vi "COD主界面.vi"() -> ()   [LabVIEW 2016]
uses:
  <vilib>/Utility/miscctls.llb/LVPointTypeDef.ctl
  <vilib>/Plasmionique/MB Master/MB_Master_Serial/MB_Master_Serial.lvclass
  F:/Program Files/National Instruments/LabVIEW 2016/vi.lib/Plasmionique/MB Master/MB_Master/MB_Master.lvclass
  <vilib>/Plasmionique/MB Master/MB Master.lvlib
panel:
  out "COD浓度（mg/L)":dbl
  out "模式选择":u16(ring) items=["COD水样测量", "COD标样核查", "COD加标回收", "COD平行样", "COD校零", "COD校标"]
  out "table 输入":string
  out "columns":string[](array[string])
  in  "保存":bool
  out "data":T1
  out "多列列表框":i32(listbox)
  in  "温度 2":dbl
  in  "恒温时间":dbl
  in  "浓度":dbl
  in  "修正系数":dbl
  in  "基本量程":enum16{"10mL", "20mL"}(ring)
  in  "水样":dbl
  in  "蒸馏水":dbl
  in  "标液":dbl
  in  "质控样":dbl
  in  "加标回收":dbl
  in  "草酸钠":dbl
  in  "高锰酸钾":dbl
  in  "硫酸":dbl
  in  "关闭":bool
  in  "零点泵计量数 2":dbl
  in  "标度泵计量数 2":dbl
  in  "标样浓度 2":dbl
  in  "unit ID":u8=1 caption="单元ID"
  out "泵1计数":dbl
  out "泵2计数":dbl
  out "泵3计数":dbl
  out "泵4计数":dbl
  out "标度滴定值":dbl
  out "零点滴定值":dbl
  in  "启动":bool
  in  "故障清除":bool
  out "排液阀故障":bool
  out "进水样超量程":bool
  out "模式（受控）":u16
  out "ORP显示":dbl
  out "温度":dbl
  out "标样核查标记":bool
  out "平行样测量":bool
  out "加标回收测量":bool
  out "质控样测量":bool
  out "待机":bool
  out "校标错误":bool
  out "校零错误":bool
  out "测量错误":bool
  out "草酸钠报警":bool
  out "高锰酸钾报警":bool
  out "加热故障":bool
  out "温控器故障":bool
  out "ORP故障":bool
  out "排液标记":bool
  out "故障标记":bool
  out "校标标记":bool
  out "校零标记":bool
  out "通讯状态":bool
  out "水样测量":bool
  in  "参数配置":bool
  in  "VISA resource name":refnum<visa-resource-name> caption="VISA资源名称"
  in  "停止 2":bool
  in  "停止":bool
  in  "单步启动":bool
  # "mV"
  # "℃"
  # "水样~加标回收"
  # "高锰酸钾"
  # "草酸钠"
  # "硫酸"
  # "基本参数设置"
  # "泵计量参数设置"
  # "校零校标结果"
  # "加热恒温温度（℃）："
  # "水样："
  # "高锰酸钾："
  # "校零结果："
  # "校零滴定值："
  # "恒温时间（分钟）："
  # "蒸馏水："
  # "草酸钠："
  # "校标结果："
  # "标度滴定值："
  # "零点泵计量值："
  # "标准液浓度（mg/L）："
  # "标液："
  # "硫酸："
  # "标度泵计量值："
  # "修正系数："
  # "质控样："
  # "标样浓度："
  # "加标回收样："
  # "基本量程（20mL可选）："
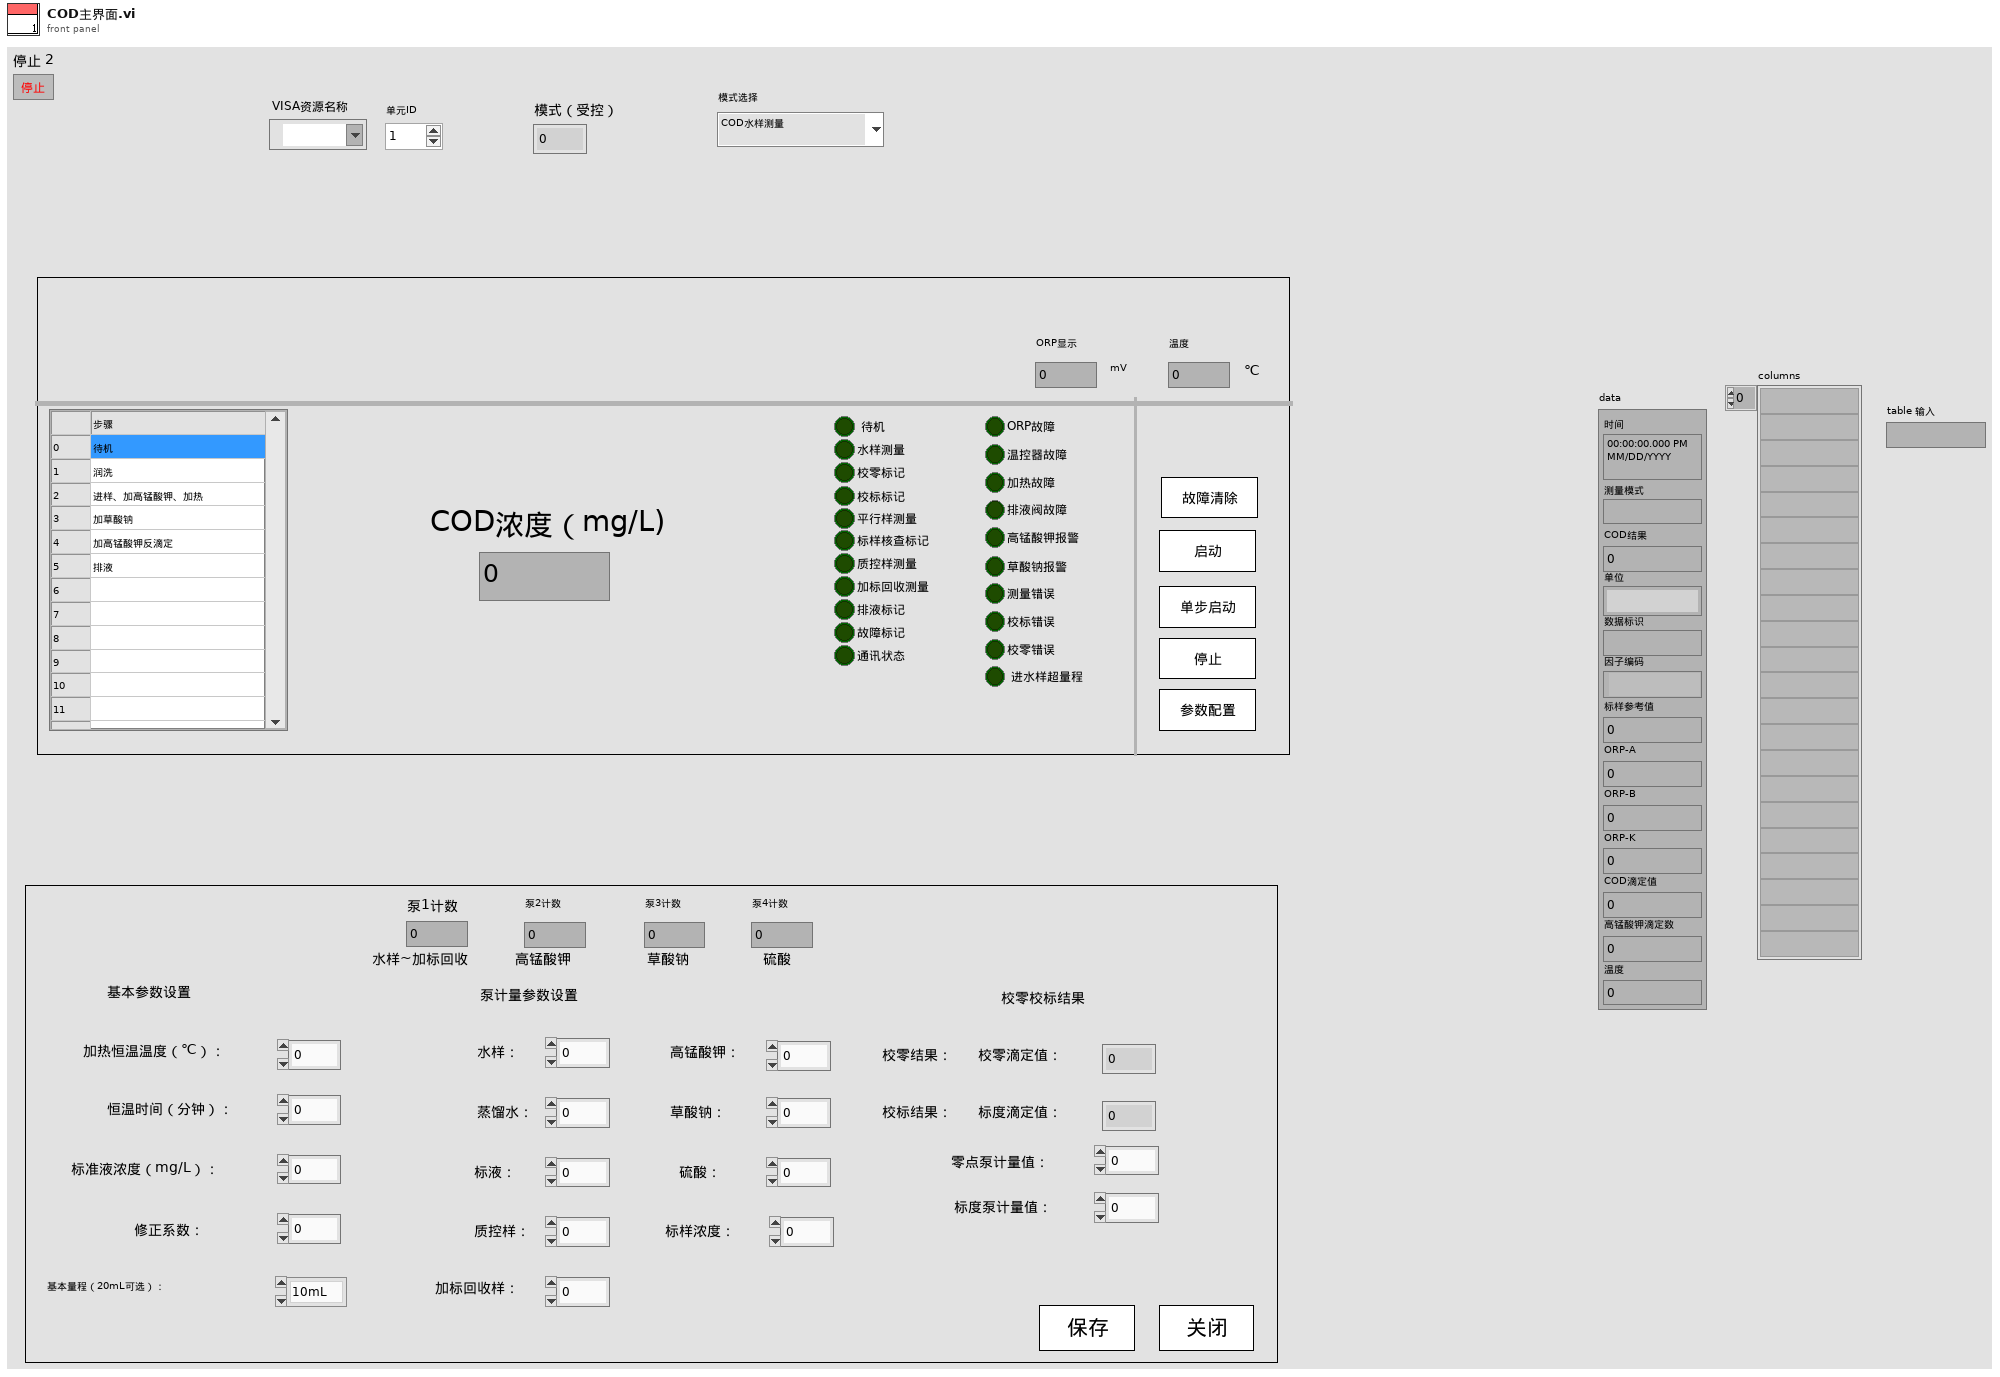
[diagram p1: front panel]
types:
  T1 = cluster{"时间":timestamp, "测量模式":string, "COD结果":sgl, "单位":string, "数据标识":string, "因子编码":string, "标样参考值":sgl, "ORP-A":sgl, "ORP-B":sgl, "ORP-K":sgl, "COD滴定值":sgl, "高锰酸钾滴定数":sgl, "温度":sgl}
  T2 = cluster{"baud rate (bps)":u32, "stop bits":u16, "parity":u16, "flow control":u16, "timeout":u32, "retries":i32}
  T3 = typedef "LVPointTypeDef.ctl" = cluster{"Horizontal":i16, "Vertical":i16}
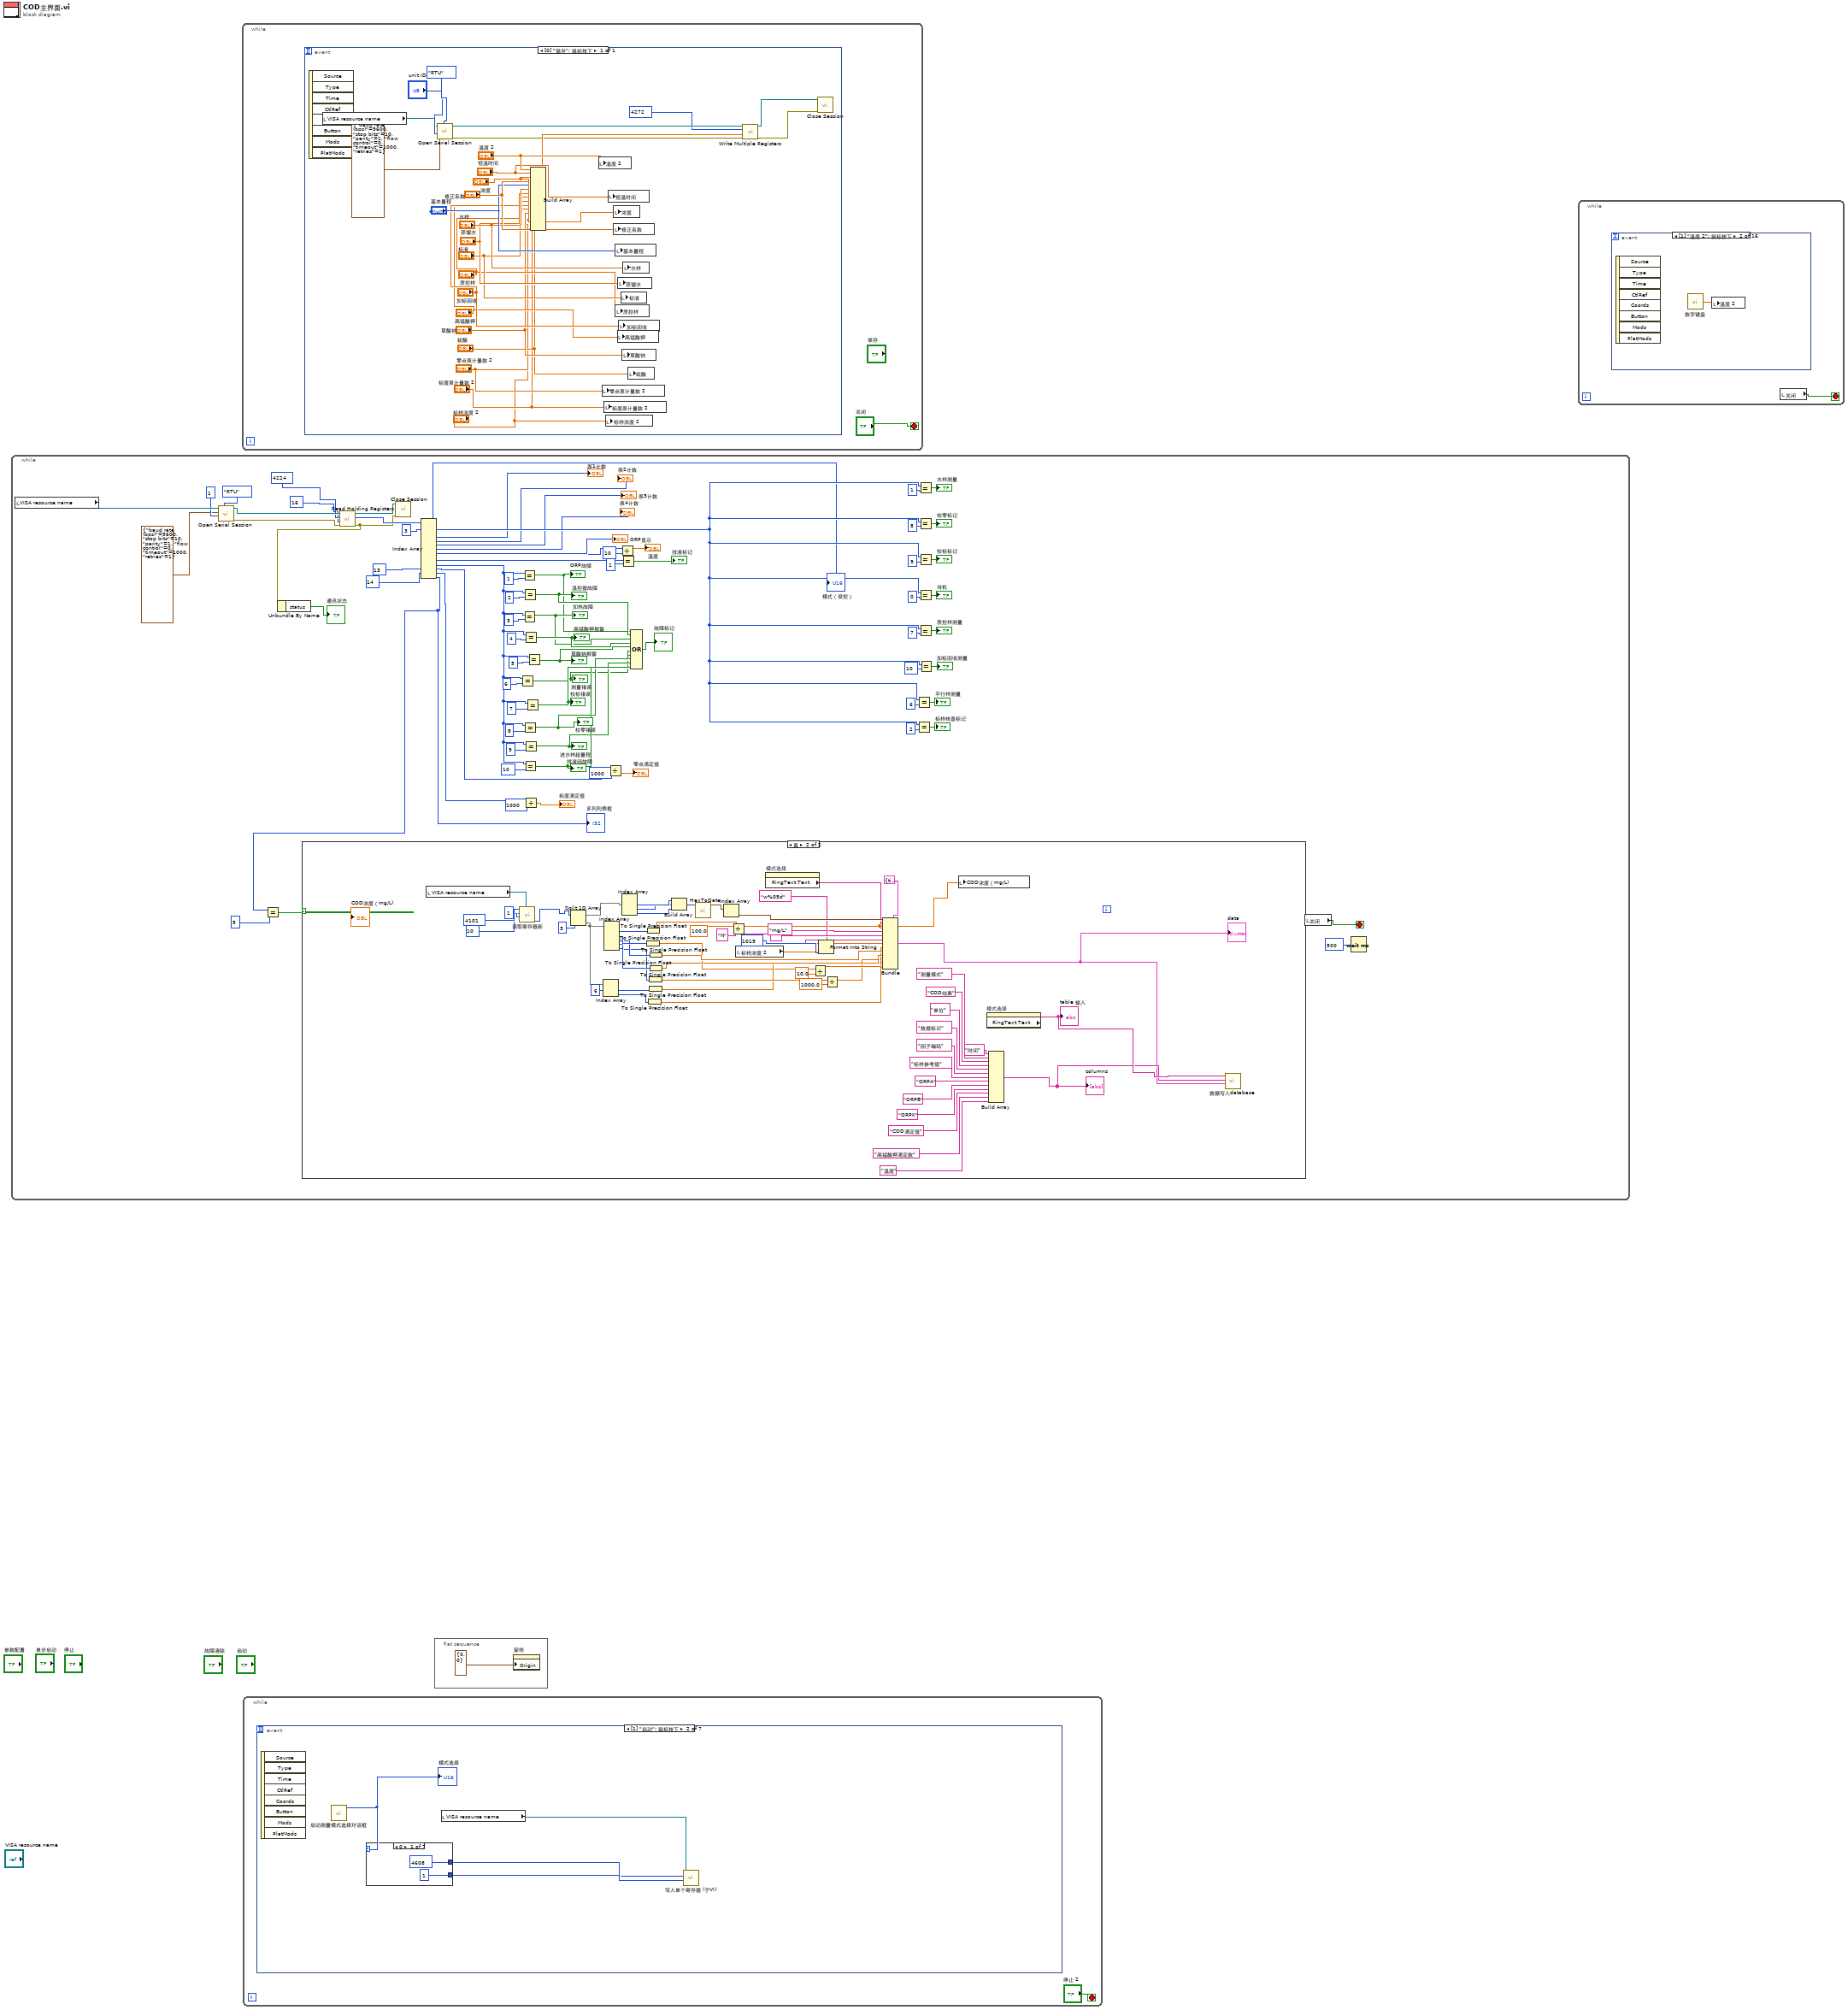
[diagram p0: block diagram]
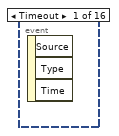
[diagram p2: hidden frame]
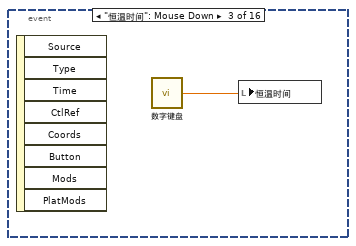
[diagram p3: hidden frame]
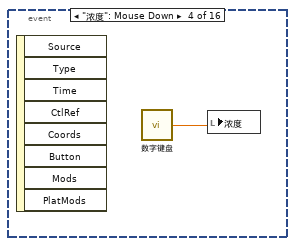
[diagram p4: hidden frame]
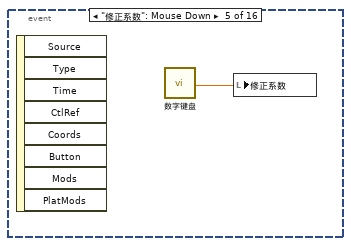
[diagram p5: hidden frame]
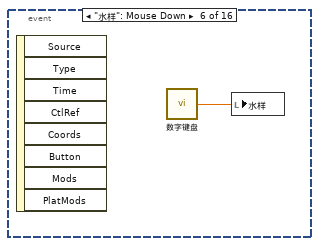
[diagram p6: hidden frame]
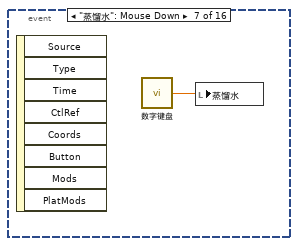
[diagram p7: hidden frame]
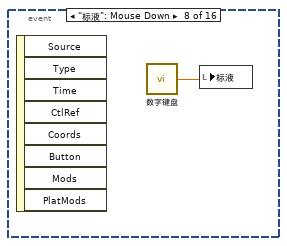
[diagram p8: hidden frame]
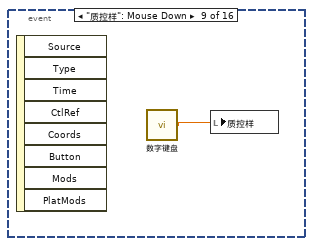
[diagram p9: hidden frame]
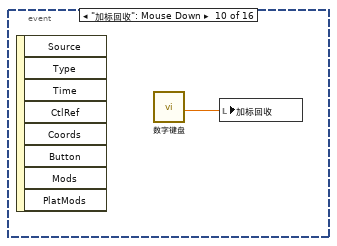
[diagram p10: hidden frame]
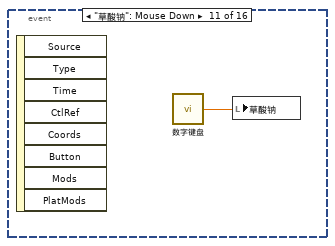
[diagram p11: hidden frame]
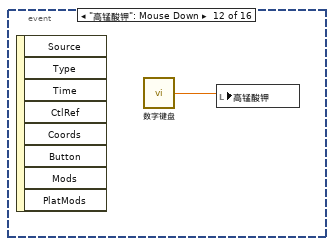
[diagram p12: hidden frame]
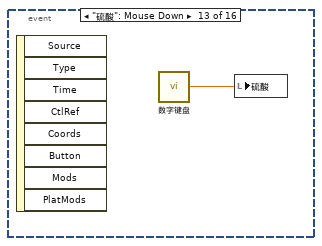
[diagram p13: hidden frame]
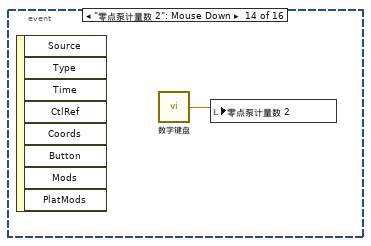
[diagram p14: hidden frame]
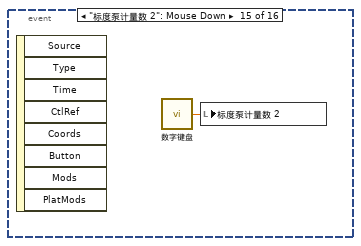
[diagram p15: hidden frame]
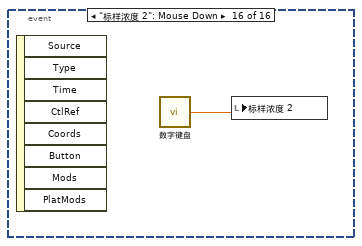
[diagram p16: hidden frame]
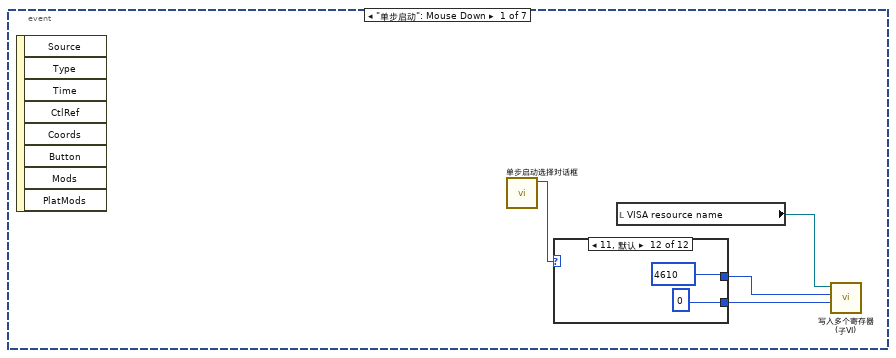
[diagram p18: hidden frame]
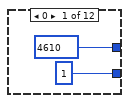
[diagram p19: hidden frame]
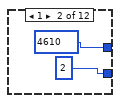
[diagram p20: hidden frame]
diagram:
  n1 = while {
    stop <- w76 stop-if-true
    n2 = local read "VISA resource name"() -> (w12:refnum<visa-resource-name>)
    n3 = call <vilib>:"Open Serial Session.vi"("Mode (RTU)"=enum16{"RTU", "ASCII"}."RTU" ("serial type"), "Slave ID"=u8 1 ("unit ID"), "Serial Config"=T2 {"baud rate (bps)"=9600, "stop bits"=10, "parity"=1, "flow control"=0, "timeout"=1000, "retries"=1}, "VISA Resource"=w12) -> ("Error out"=w11:errorcluster, "MB_Serial session"=w10:refnum<class "MB_Master_Serial.lvclass">)  [unwired: 6 in]
    n4 = call <vilib>:"Read Holding Registers.vi"("error in (no error)"=w11, "quantity"=u16 16 ("number of holding registers"), "starting address"=u16 4224, "MB session in"=w10) -> ("error out"=w2:errorcluster, "Registers"=w4:u16[], "MB session out"=w3:refnum<class "MB_Master_Serial.lvclass">)  [unwired: 5 in]
    n5 = Unbundle By Name(w2) -> ("status"=→"通讯状态":bool)
    n6 = call-dynamic "Close Session.vi"("error in (no error)"=w2, "MB_Serial session"=w3) -> ()  [unwired: 9 in, 1 out]
    n7 = Index Array(array=w4, index #1=3 ("索引"), index #11=13 ("索引"), index #12=14 ("索引")) -> (element #1=w56:u16, element #2=→"模式（受控）":u16, element #3=→"泵1计数":u16, element #4=→"泵2计数":u16, element #5=→"泵3计数":u16, element #6=→"泵4计数":u16, element #7=→"ORP显示":u16, element #8=w49:u16, element #9=w47:u16, element #10=w24:u16, element #11=w19:u16, element #12=w16:u16, element #13=w22:u16)  [unwired: 10 in]
    "多列列表框" <- w22
    n8 = Equal?(x=w22, y=u16 5) -> (x = y?=w74:bool)
    n9 = case shown="真" w74 {
      frame False {
      }
      frame True {
        n10 = local read "VISA resource name"() -> (w82:refnum<visa-resource-name>)
        n11 = call "读取寄存器新.vi"("VISA Resource"=w82, "Slave ID"=u8 1 ("unit ID"), "quantity"=u16 10 ("number of holding registers"), "starting address"=u16 4101) -> ("Registers"=w83:u16[])  [unwired: 7 in]
        n12 = Split 1D Array(array=w83, index=3 ("索引")) -> (first subarray=w135:u16[], second subarray=w123:u16[])
        n13 = Index Array(array=w123, index #1=6 ("索引")) -> (element #1=w121:u16, element #2=w120:u16)  [unwired: 1 in]
        n14 = Index Array(array=w123) -> (element #1=w128:u16, element #2=w127:u16, element #3=w126:u16, element #4=w125:u16, element #5=w124:u16)  [unwired: 5 in]
        n15 = Index Array(array=w135) -> (element #1=w133:u16, element #2=w132:u16, element #3=w131:u16)  [unwired: 3 in]
        n16 = To Single Precision Float(number=w127) -> (single precision float=w91:sgl)
        n17 = To Single Precision Float(number=w128) -> (single precision float=w119:sgl)
        n18 = To Single Precision Float(number=w120) -> (single precision float=w109:sgl)
        n19 = To Single Precision Float(number=w124) -> (single precision float=w111:sgl)
        n20 = To Single Precision Float(number=w121) -> (single precision float=w110:sgl)
        n21 = To Single Precision Float(number=w126) -> (single precision float=w113:sgl)
        n22 = To Single Precision Float(number=w125) -> (single precision float=w112:sgl)
        n23 = Build Array(w133, w132, w131) -> (w130:u16[])
        n24 = call "HexToDate.vi"("数组"=w130) -> ("DATE"=w134:timestamp[])  [unwired: 10 in]
        n25 = Index Array(array=w134) -> (element=w129:timestamp)  [unwired: 1 in]
        n26 = Divide(x=w119, y=sgl 100.0) -> (x/y=w78:sgl)
        n27 = local read "标样浓度 2"() -> (w114:dbl)
        n28 = property on="模式选择" class="Ring (严格)"() -> ("RingText.Text"=w95:string)  [unwired: 2 in, 2 out]
        n29 = Divide(x=w91, y=sgl 10.0) -> (x/y=w92:sgl)
        n30 = Format Into String(format string="w%05d" ("格式字符串"), u32 1019 ("因子编码")) -> (resulting string=w115:string)  [unwired: 2 in, 1 out]
        n31 = Divide(x=w111, y=sgl 1000.0) -> (x/y=w89:sgl)
        n32 = Bundle(cluster=T1 {"时间"=timestamp(0 s since 1904-01-01), "测量模式"="COD水样测量", "COD结果"=0.0, "单位"="mg/L", "数据标识"="N", "因子编码"="w01019", "标样参考值"=0.0, "ORP-A"=0.0, "ORP-B"=0.0, "ORP-K"=0.0, "COD滴定值"=0.0, "高锰酸钾滴定数"=0.0, "温度"=0.0} ("data"), "时间"=w129, "测量模式"=w95, "COD结果"=w78, "单位"="mg/L", "数据标识"="N", "因子编码"=w115, "标样参考值"=w114, "ORP-A"=w92, "ORP-B"=w113, "ORP-K"=w112, "COD滴定值"=w89, "高锰酸钾滴定数"=w110, "温度"=w109) -> (w80:T1)
        "data" <- w80
        n33 = local write "COD浓度（mg/L)"(w78) -> ()
        n34 = property on="模式选择" class="Ring (严格)"() -> ("RingText.Text"=w94:string)  [unwired: 2 in, 2 out]
        "table 输入" <- w94
        n35 = Build Array("时间", "测量模式", "COD结果", "单位", "数据标识", "因子编码", "标样参考值", "ORPA", "ORPB", "ORPK", "COD滴定值", "高锰酸钾滴定数", "温度") -> (w93:string[])
        "columns" <- w93
        n36 = call "数据写入database.vi"("data"=w80, "columns"=w93, "table"=w94) -> ()  [unwired: 9 in]
      }
    }
    n37 = Equal?(x=w24, y=u16 6) -> (x = y?=w40:bool)
    "测量错误" <- w40
    n38 = Equal?(x=w24, y=u16 1) -> (x = y?=w35:bool)
    "ORP故障" <- w35
    n39 = Equal?(x=w24, y=u16 3) -> (x = y?=w37:bool)
    "加热故障" <- w37
    n40 = Equal?(x=w24, y=u16 2) -> (x = y?=w36:bool)
    "温控器故障" <- w36
    n41 = Equal?(x=w24, y=u16 8) -> (x = y?=w42:bool)
    "校零错误" <- w42
    n42 = Equal?(x=w24, y=u16 10) -> (x = y?=w44:bool)
    "排液阀故障" <- w44
    n43 = Equal?(x=w24, y=u16 4) -> (x = y?=w38:bool)
    "高锰酸钾报警" <- w38
    n44 = Equal?(x=w24, y=u16 9) -> (x = y?=w43:bool)
    "进水样超量程" <- w43
    n45 = Divide(x=w16, y=u16 1000) -> (x/y=→"标度滴定值":dbl)
    n46 = Equal?(x=w24, y=u16 7) -> (x = y?=w41:bool)
    "校标错误" <- w41
    n47 = Equal?(x=w24, y=u16 5) -> (x = y?=w39:bool)
    "草酸钠报警" <- w39
    n48 = Divide(x=w19, y=u16 1000) -> (x/y=→"零点滴定值":dbl)
    n49 = Divide(x=w49, y=u16 10) -> (x/y=→"温度":dbl)
    n50 = Equal?(x=w47, y=u16 1) -> (x = y?=→"排液标记":bool)
    n51 = Compound Arithmetic op=OR ("复合运算")(w35, w36, w37, w38, w39, w40, w41, w42, w43, w44) -> (→"故障标记":bool)
    n52 = Equal?(x=w56, y=u16 6) -> (x = y?=→"平行样测量":bool)
    n53 = Equal?(x=w56, y=u16 2) -> (x = y?=→"标样核查标记":bool)
    n54 = Equal?(x=w56, y=u16 1) -> (x = y?=→"水样测量":bool)
    n55 = Equal?(x=w56, y=u16 8) -> (x = y?=→"校零标记":bool)
    n56 = Equal?(x=w56, y=u16 9) -> (x = y?=→"校标标记":bool)
    n57 = Equal?(x=w56, y=u16 0) -> (x = y?=→"待机":bool)
    n58 = Equal?(x=w56, y=u16 7) -> (x = y?=→"质控样测量":bool)
    n59 = Equal?(x=w56, y=u16 10) -> (x = y?=→"加标回收测量":bool)
    n60 = local read "关闭"() -> (w76:bool)
    n61 = Wait (ms)(milliseconds to wait=u32 500 ("等待时间（毫秒）")) -> ()  [unwired: 1 out]
  }
  n62 = while {
    stop <- "关闭" stop-if-true
    n63 = event shown="[0] \"保存\": 鼠标按下" {
      selector: _ -> [_]
      dyn-events: _ -> [_]
      timeout: _ -> [_]
      event "保存": Mouse Down {
        n64 = event-data() -> ()  [unwired: 1 in, 8 out]
        n65 = local read "VISA resource name"() -> (w145:refnum<visa-resource-name>)
        n66 = call <vilib>:"Open Serial Session.vi"("Mode (RTU)"=enum16{"RTU", "ASCII"}."RTU" ("serial type"), "Slave ID"="unit ID", "Serial Config"=T2 {"baud rate (bps)"=9600, "stop bits"=10, "parity"=1, "flow control"=0, "timeout"=1000, "retries"=1}, "VISA Resource"=w145) -> ("Error out"=w140:errorcluster, "MB_Serial session"=w143:refnum<class "MB_Master_Serial.lvclass">)  [unwired: 6 in]
        n67 = Build Array("温度 2", "恒温时间", "浓度", "修正系数", "基本量程", "水样", "蒸馏水", "标液", "质控样", "加标回收", "高锰酸钾", "草酸钠", "硫酸", "零点泵计量数 2", "标度泵计量数 2", "标样浓度 2") -> (w141:dbl[])
        n68 = local write "温度 2"("温度 2") -> ()
        n69 = local write "零点泵计量数 2"("零点泵计量数 2") -> ()
        n70 = local write "标度泵计量数 2"("标度泵计量数 2") -> ()
        n71 = local write "标样浓度 2"("标样浓度 2") -> ()
        n72 = local write "恒温时间"("恒温时间") -> ()
        n73 = local write "浓度"("浓度") -> ()
        n74 = local write "修正系数"("修正系数") -> ()
        n75 = local write "基本量程"("基本量程") -> ()
        n76 = local write "质控样"("质控样") -> ()
        n77 = local write "高锰酸钾"("高锰酸钾") -> ()
        n78 = local write "蒸馏水"("蒸馏水") -> ()
        n79 = local write "加标回收"("加标回收") -> ()
        n80 = local write "标液"("标液") -> ()
        n81 = local write "草酸钠"("草酸钠") -> ()
        n82 = local write "水样"("水样") -> ()
        n83 = local write "硫酸"("硫酸") -> ()
        n84 = call <vilib>:"Write Multiple Registers.vi"("error in (no error)"=w140, "values"=w141, "starting address"=u16 4272, "MB session in"=w143) -> ("error out"=w139:errorcluster, "MB session out"=w138:refnum<class "MB_Master_Serial.lvclass">)  [unwired: 6 in]
        n85 = call-dynamic "Close Session.vi"("error in (no error)"=w139, "MB_Serial session"=w138) -> ()  [unwired: 9 in, 1 out]
      }
    }
  }
  n86 = while {
    stop <- "停止 2" stop-if-true
    n87 = event shown="[1] \"启动\": 鼠标按下" {
      selector: _ -> [_ _ _ _ _ _ _]
      dyn-events: _ -> [_ _ _ _ _ _ _]
      timeout: _ -> [_ _ _ _ _ _ _]
      event "单步启动": Mouse Down {
        n88 = event-data() -> ()  [unwired: 1 in, 8 out]
        n89 = call "单步启动选择对话框.vi"() -> ("启动选择 2"=w168:u16)  [unwired: 11 in]
        n90 = case shown="11, 默认" w168 {
          tunnel: [u16 4610 ("address") u16 4610 ("address") u16 4610 ("address") u16 4610 ("address") u16 4610 ("address") u16 4610 ("address") u16 4610 ("address") u16 4610 ("address") u16 4610 ("address") u16 4610 ("address") u16 4610 ("address") u16 4610 ("address")] -> w166
          tunnel: [u16 1 ("address") u16 2 ("address") u16 3 ("address") u16 4 ("address") u16 5 ("address") u16 6 ("address") u16 7 ("address") u16 8 ("address") u16 9 ("holding register value") u16 10 ("holding register value") u16 11 ("holding register value") u16 0 ("address")] -> w165
          frame 0 {
          }
          frame 1 {
          }
          frame 2 {
          }
          frame 3 {
          }
          frame 4 {
          }
          frame 5 {
          }
          frame 6 {
          }
          frame 7 {
          }
          frame 8 {
          }
          frame 9 {
          }
          frame 10 {
          }
          frame 11, Default {
          }
        }
        n91 = local read "VISA resource name"() -> (w167:refnum<visa-resource-name>)
        n92 = call "写入多个寄存器 (子VI).vi"("holding register value"=w165, "address"=w166, "VISA resource name"=w167) -> ()  [unwired: 8 in, 1 out]
      }
      event "启动": Mouse Down {
        n93 = event-data() -> ()  [unwired: 1 in, 8 out]
        n94 = call "启动测量模式选择对话框.vi"() -> ("启动选择 2"=w196:u16)  [unwired: 11 in]
        "模式选择" <- w196
        n95 = case shown="0" w196 {
          tunnel: [u16 4608 ("address") u16 4608 ("address") u16 4608 ("address") u16 4608 ("address") u16 4608 ("address") u16 4608 ("address") u16 4608 ("address")] -> w194
          tunnel: [u16 1 ("address") u16 2 ("address") u16 7 ("address") u16 6 ("address") u16 8 ("address") u16 9 ("address") u16 0 ("address")] -> w193
          frame 0 {
          }
          frame 1 {
          }
          frame 2 {
          }
          frame 3 {
          }
          frame 4 {
          }
          frame 5 {
          }
          frame 6, Default {
          }
        }
        n96 = local read "VISA resource name"() -> (w195:refnum<visa-resource-name>)
        n97 = call "写入单个寄存器 (子VI).vi"("值"=w194, "address"=w193, "VISA引用句柄输入"=w195) -> ()  [unwired: 9 in]
      }
      event "停止": Mouse Down {
        n98 = event-data() -> ()  [unwired: 1 in, 8 out]
        n99 = local read "VISA resource name"() -> (w213:refnum<visa-resource-name>)
        n100 = call "写入单个寄存器 (子VI).vi"("值"=u16 11 ("holding register value"), "address"=u16 4608, "VISA引用句柄输入"=w213) -> ()  [unwired: 9 in]
      }
      event "参数配置": Mouse Down {
        n101 = event-data() -> ()  [unwired: 1 in, 8 out]
        n102 = property on="窗格" class="Pane"("Origin"=T3 {"Horizontal"=0, "Vertical"=600} ("原点")) -> ()  [unwired: 2 in, 2 out]
      }
      event "关闭": Mouse Down {
        n103 = event-data() -> ()  [unwired: 1 in, 8 out]
        n104 = property on="窗格" class="Pane"("Origin"=T3 {"Horizontal"=0, "Vertical"=0} ("原点")) -> ()  [unwired: 2 in, 2 out]
      }
      event Timeout {
        n105 = event-data() -> ()  [unwired: 1 in, 3 out]
      }
      event "故障清除": Mouse Down {
        n106 = event-data() -> ()  [unwired: 1 in, 8 out]
        n107 = local read "VISA resource name"() -> (w218:refnum<visa-resource-name>)
        n108 = call "写入单个寄存器 (子VI).vi"("值"=u16 1 ("holding register value"), "address"=u16 4611, "VISA引用句柄输入"=w218) -> ()  [unwired: 9 in]
      }
    }
  }
  n109 = flat-sequence {
    frame #0 {
      n110 = property on="窗格" class="Pane"("Origin"=T3 {"Horizontal"=0, "Vertical"=0} ("原点")) -> ()  [unwired: 2 in, 2 out]
    }
  }
  n111 = while {
    stop <- w220 stop-if-true
    n112 = event shown="[1] \"温度 2\": 鼠标按下" {
      selector: _ -> [_ _ _ _ _ _ _ _ _ _ _ _ _ _ _ _]
      dyn-events: _ -> [_ _ _ _ _ _ _ _ _ _ _ _ _ _ _ _]
      timeout: _ -> [_ _ _ _ _ _ _ _ _ _ _ _ _ _ _ _]
      event Timeout {
        n113 = event-data() -> ()  [unwired: 1 in, 3 out]
      }
      event "温度 2": Mouse Down {
        n114 = event-data() -> ()  [unwired: 1 in, 8 out]
        n115 = call "数字键盘.vi"() -> ("NewNumber"=w221:sgl)  [unwired: 1 in]
        n116 = local write "温度 2"(w221) -> ()
      }
      event "恒温时间": Mouse Down {
        n117 = event-data() -> ()  [unwired: 1 in, 8 out]
        n118 = call "数字键盘.vi"() -> ("NewNumber"=w222:sgl)  [unwired: 1 in]
        n119 = local write "恒温时间"(w222) -> ()
      }
      event "浓度": Mouse Down {
        n120 = event-data() -> ()  [unwired: 1 in, 8 out]
        n121 = call "数字键盘.vi"() -> ("NewNumber"=w223:sgl)  [unwired: 1 in]
        n122 = local write "浓度"(w223) -> ()
      }
      event "修正系数": Mouse Down {
        n123 = event-data() -> ()  [unwired: 1 in, 8 out]
        n124 = call "数字键盘.vi"() -> ("NewNumber"=w224:sgl)  [unwired: 1 in]
        n125 = local write "修正系数"(w224) -> ()
      }
      event "水样": Mouse Down {
        n126 = event-data() -> ()  [unwired: 1 in, 8 out]
        n127 = call "数字键盘.vi"() -> ("NewNumber"=w225:sgl)  [unwired: 1 in]
        n128 = local write "水样"(w225) -> ()
      }
      event "蒸馏水": Mouse Down {
        n129 = event-data() -> ()  [unwired: 1 in, 8 out]
        n130 = call "数字键盘.vi"() -> ("NewNumber"=w226:sgl)  [unwired: 1 in]
        n131 = local write "蒸馏水"(w226) -> ()
      }
      event "标液": Mouse Down {
        n132 = event-data() -> ()  [unwired: 1 in, 8 out]
        n133 = call "数字键盘.vi"() -> ("NewNumber"=w227:sgl)  [unwired: 1 in]
        n134 = local write "标液"(w227) -> ()
      }
      event "质控样": Mouse Down {
        n135 = event-data() -> ()  [unwired: 1 in, 8 out]
        n136 = call "数字键盘.vi"() -> ("NewNumber"=w228:sgl)  [unwired: 1 in]
        n137 = local write "质控样"(w228) -> ()
      }
      event "加标回收": Mouse Down {
        n138 = event-data() -> ()  [unwired: 1 in, 8 out]
        n139 = call "数字键盘.vi"() -> ("NewNumber"=w229:sgl)  [unwired: 1 in]
        n140 = local write "加标回收"(w229) -> ()
      }
      event "草酸钠": Mouse Down {
        n141 = event-data() -> ()  [unwired: 1 in, 8 out]
        n142 = call "数字键盘.vi"() -> ("NewNumber"=w230:sgl)  [unwired: 1 in]
        n143 = local write "草酸钠"(w230) -> ()
      }
      event "高锰酸钾": Mouse Down {
        n144 = event-data() -> ()  [unwired: 1 in, 8 out]
        n145 = call "数字键盘.vi"() -> ("NewNumber"=w231:sgl)  [unwired: 1 in]
        n146 = local write "高锰酸钾"(w231) -> ()
      }
      event "硫酸": Mouse Down {
        n147 = event-data() -> ()  [unwired: 1 in, 8 out]
        n148 = call "数字键盘.vi"() -> ("NewNumber"=w232:sgl)  [unwired: 1 in]
        n149 = local write "硫酸"(w232) -> ()
      }
      event "零点泵计量数 2": Mouse Down {
        n150 = event-data() -> ()  [unwired: 1 in, 8 out]
        n151 = call "数字键盘.vi"() -> ("NewNumber"=w233:sgl)  [unwired: 1 in]
        n152 = local write "零点泵计量数 2"(w233) -> ()
      }
      event "标度泵计量数 2": Mouse Down {
        n153 = event-data() -> ()  [unwired: 1 in, 8 out]
        n154 = call "数字键盘.vi"() -> ("NewNumber"=w234:sgl)  [unwired: 1 in]
        n155 = local write "标度泵计量数 2"(w234) -> ()
      }
      event "标样浓度 2": Mouse Down {
        n156 = event-data() -> ()  [unwired: 1 in, 8 out]
        n157 = call "数字键盘.vi"() -> ("NewNumber"=w235:sgl)  [unwired: 1 in]
        n158 = local write "标样浓度 2"(w235) -> ()
      }
    }
    n159 = local read "关闭"() -> (w220:bool)
  }
